vi "Close Control.vi"(8 "error in (no error)":errorcluster, 11 "D_Datagrid in":refnum<class "D_Datagrid.lvclass">) -> (0 "error out":errorcluster, 3 "D_Datagrid out":refnum<class "D_Datagrid.lvclass">)   [LabVIEW 2023, in "D Datagrid Library.lvlib" / "D_Datagrid.lvclass"]
doc: "The <b>Close Control VI</b> is a dynamic dispatch VI that must be used in the cleanup of portion of the calling code before ending.\n\nIt should be overwritten if the QControl Class needs to do any uninitialization or closing of references.\n\nIf overwritten, the <b>Call Parent Method</b> must be called in order to cleanup the control reference, close running <b>Event Handler VI</b> (if there is one), and release the State Data DVR (if there is one).\n<b> </b> <b> </b>\n©2016 Q Software Innovations, LLC (QSI)\nwritten by Quentin Alldredge\nproduced in LabVIEW 2015\n\nsupport@qsoftwareinnovations.com\nwww.qsoftwareinnovations.com\n\nAll rights reserved.\n\nRedistribution and use in source and binary forms, with or without modification, are permitted provided that the following conditions are met:\n\n * Redistributions of source code must retain the above copyright notice, this list of conditions and the following disclaimer.\n * Redistributions in binary form must reproduce the above copyright notice, this list of conditions and the following disclaimer in the documentation and/or other materials provided with the distribution.\n * Neither the name of Q Software Innovations, LLC. nor the names of its contributors may be used to endorse or promote products derived from this software without specific prior written permission.\n\nTHIS SOFTWARE IS PROVIDED BY THE COPYRIGHT HOLDERS AND CONTRIBUTORS \"AS IS\" AND ANY EXPRESS OR IMPLIED WARRANTIES, INCLUDING, BUT NOT LIMITED TO, THE IMPLIED WARRANTIES OF MERCHANTABILITY AND FITNESS FOR A PARTICULAR PURPOSE ARE DISCLAIMED. IN NO EVENT SHALL THE COPYRIGHT OWNER OR CONTRIBUTORS BE LIABLE FOR ANY DIRECT, INDIRECT, INCIDENTAL, SPECIAL, EXEMPLARY, OR CONSEQUENTIAL DAMAGES (INCLUDING, BUT NOT LIMITED TO, PROCUREMENT OF SUBSTITUTE GOODS OR SERVICES; LOSS OF USE, DATA, OR PROFITS; OR BUSINESS INTERRUPTION) HOWEVER CAUSED AND ON ANY THEORY OF LIABILITY, WHETHER IN CONTRACT, STRICT LIABILITY, OR TORT (INCLUDING NEGLIGENCE OR OTHERWISE) ARISING IN ANY WAY OUT OF THE USE OF THIS SOFTWARE, EVEN IF ADVISED OF THE POSSIBILITY OF SUCH DAMAGE."
uses:
  D_Datagrid.lvclass
  D_Datagrid.lvclass/D_Datagrid.ctl
  <vilib>/QSI/QControls/QControl Classes/Table/Table.lvclass
  Scrolling behavior.ctl
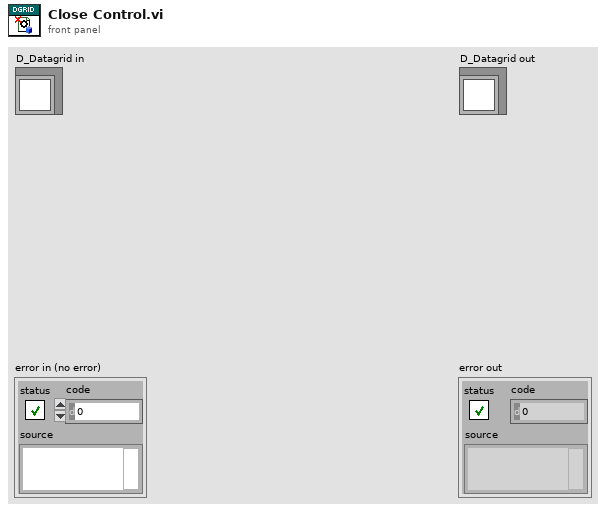
[diagram p1: front panel]
types:
  T1 = typedef "D Datagrid Library.lvlib/D_Datagrid.lvclass/Scrolling behavior.ctl" = enum16{"Default", "Locked", "Displayed items only"}
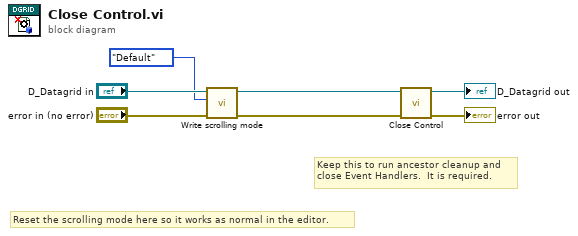
[diagram p0: block diagram]
diagram:
  # "Reset the scrolling mode here so it works as normal in the editor."
  # "Keep this to run ancestor cleanup and\nclose Event Handlers.  It is required."
  n1 = call "Write scrolling mode.vi"("error in (no error)"="error in (no error)", "Scrolling mode"=Scrolling_behavior."Default", "D_Datagrid in"="D_Datagrid in") -> ("error out"=w1:errorcluster, "D_Datagrid out"=w2:refnum<class "D_Datagrid.lvclass">)  [unwired: 7 in]
  n2 = call-parent "Close Control.vi"("error in (no error)"=w1, "Control in"=w2) -> ("error out"=→"error out":errorcluster, "Control out"=→"D_Datagrid out":refnum<class "D_Datagrid.lvclass">)  [unwired: 8 in]
